vi "changePath.vi"(11 "Local Saving in (h)":path) -> (2 "change (h)":bool, 3 "Local Saving out (h)":path)   [LabVIEW 2013]
panel:
  in  "Chancel":bool
  in  "OK Button":bool
  in  "Local Saving Path":path
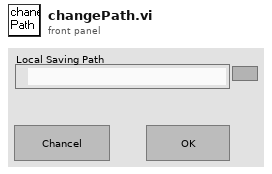
[diagram p1: front panel]
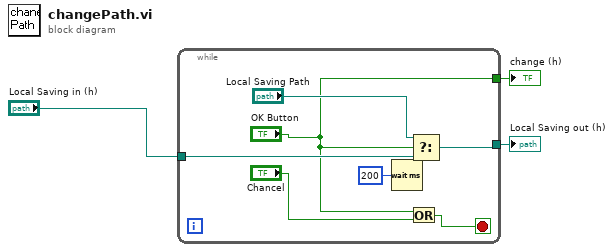
[diagram p0: block diagram]
diagram:
  n1 = while {
    tunnel: "Local Saving in (h)" -> [w7]
    tunnel: [w6] -> w2
    tunnel: ["OK Button"] -> w1
    stop <- w9 stop-if-true
    n2 = Wait (ms)(milliseconds to wait=u32 200) -> ()  [unwired: 1 out]
    n3 = Or(x="OK Button", y="Chancel") -> (x .or. y?=w9:bool)
    n4 = Select(t="Local Saving Path", s="OK Button", f=w7) -> (s? t:f=w6:path)
  }
  "Local Saving out (h)" <- w2
  "change (h)" <- w1
